vi "ChangeAssignedShortcut.vi"(7 "QDKS Info":T1[](array[typedef]), 8 "error in (no error)":errorcluster, 10 "Key":string, 11 "QD":string) -> (0 "error out":errorcluster)   [LabVIEW 2020, in "NEVSTOP QD Shortcuts.lvlib"]
uses:
  NEVSTOP QD Shortcuts.lvlib
  <resource>/dialog/QuickDrop/QuickDrop QDKS Info.ctl
  <resource>/dialog/lvconfig.llb/LV Config Write String.vi
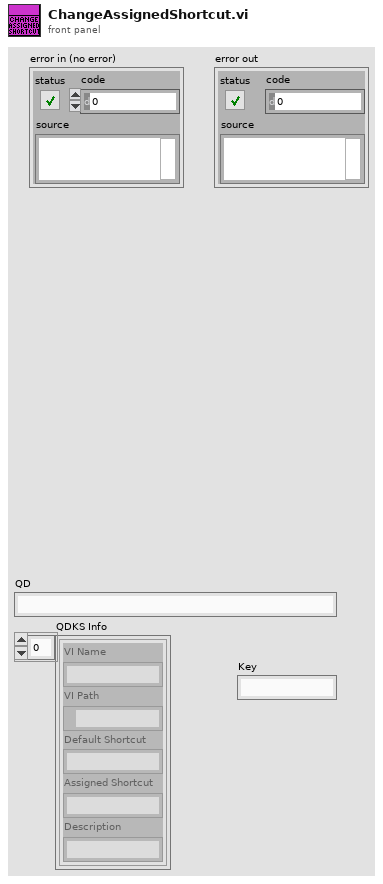
[diagram p1: front panel]
types:
  T1 = typedef "QuickDrop QDKS Info.ctl" = cluster{"VI Name":string, "VI Path":path, "Default Shortcut":string, "Assigned Shortcut":string, "Description":string}
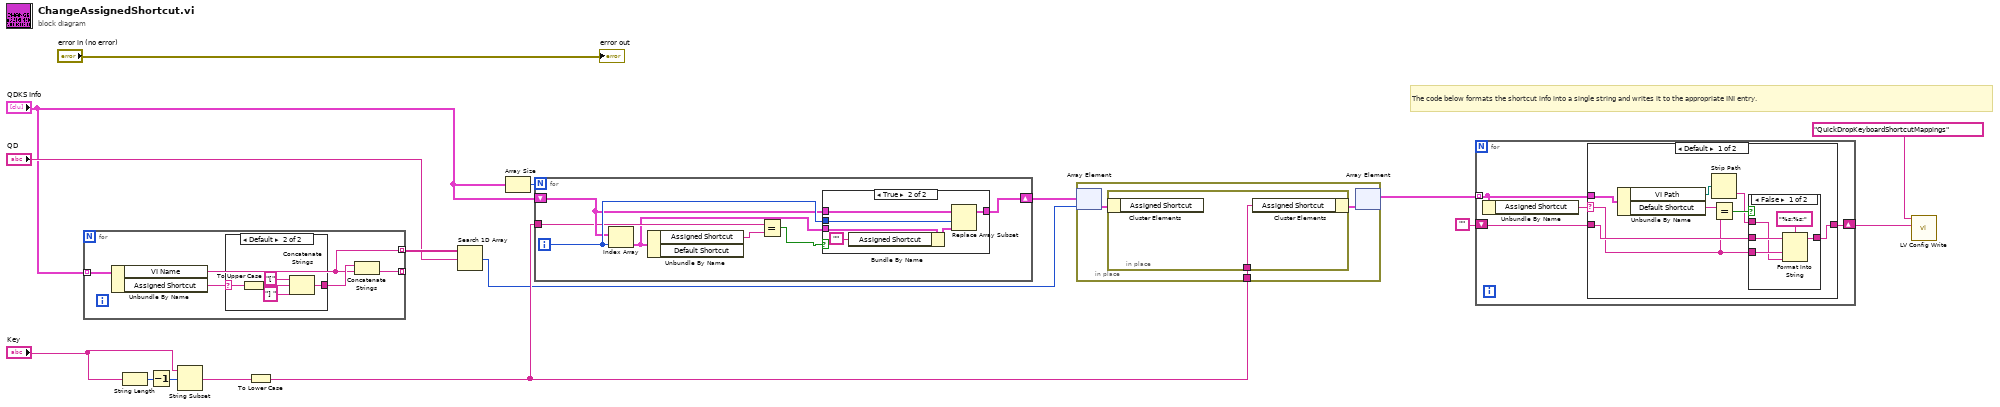
[diagram p0: block diagram]
diagram:
  # "The code below formats the shortcut info into a single string and writes it to the appropriate INI entry."
  n1 = for {
    tunnel: "QDKS Info" -> [w21] mode=indexing
    tunnel: [w20] -> _ mode=indexing
    tunnel: [w17] -> w7 mode=indexing
    n2 = Unbundle By Name(w21) -> ("VI Name"=w17:string, "Assigned Shortcut"=w19:string)
    n3 = case shown="Default" w19 {
      selector: w19 -> [_ w26]
      tunnel: [_ w25] -> w18
      frame "" {
      }
      frame Default {
        n4 = To Upper Case(1:w26) -> (0:w22:string)
        n5 = Concatenate Strings("[" ("string"), w22, "] " ("string")) -> (w25:string)
      }
    }
    n6 = Concatenate Strings(w18, w17) -> (w20:string)
  }
  n7 = String Length(string="Key") -> (length=w15:i32)
  n8 = Decrement(x=w15) -> (x-1=w14:i32)
  n9 = String Subset(string="Key", offset (0)=w14) -> (substring=w13:string)  [unwired: 1 in]
  n10 = To Lower Case(string=w13) -> (all lower case string=w11:string)
  n11 = Search 1D Array(1D array=w7, element="QD") -> (index of element=w5:i32)  [unwired: 1 in]
  n12 = Array Size(array="QDKS Info") -> (size(s)=w12:i32)
  n13 = for {
    N: w12 -> [_]
    shift-right: [w31] -> w2
    shift-left: "QDKS Info" -> [w32]
    tunnel: w11 -> [w30]
    i -> [w33]
    n14 = Index Array(array=w32, index=w33) -> (element=w28:T1)
    n15 = Unbundle By Name(w28) -> ("Assigned Shortcut"=w29:string)  [unwired: 1 out]
    n16 = Equal?(x=w30, y=w29) -> (x = y?=w27:bool)
    n17 = case shown="True" w27 {
      tunnel: w32 -> [w34 w40]
      tunnel: [w34 w39] -> w31
      tunnel: w33 -> [_ w38]
      tunnel: w28 -> [_ w37]
      frame False {
      }
      frame True {
        n18 = Bundle By Name(cluster=w37, "Assigned Shortcut"="") -> (w36:T1)
        n19 = Replace Array Subset(array=w40, new element=w36, index=w38) -> (w39:T1[])
      }
    }
  }
  n20 = in-place {
    in-place-border: w11 -> [w41]
    n21 = in-place-array #1(w2, w5) -> (w43:T1)
    n22 = in-place {
      in-place-border: w41 -> [w44]
      n23 = in-place-cluster #2(w43) -> ()  [unwired: 1 out]
      n24 = in-place-cluster #2("Assigned Shortcut"=w44) -> (w42:T1)
    }
    n25 = in-place-array #1(w42) -> (w1:T1[])  [unwired: 1 out]
  }
  n26 = for {
    tunnel: w1 -> [w45] mode=indexing
    shift-right: [w46] -> w9
    shift-left: "" -> [w47]
    n27 = Unbundle By Name(w45) -> ("Assigned Shortcut"=w48:string)
    n28 = case shown="Default" w48 {
      selector: w48 -> [w52 _]
      tunnel: w47 -> [w54 w63]
      tunnel: [w55 w63] -> w46
      tunnel: w45 -> [w56 _]
      frame Default {
        n29 = Unbundle By Name(w56) -> ("VI Path"=w50:path, "Default Shortcut"=w53:string)
        n30 = Strip Path(path=w50) -> (name=w49:string)  [unwired: 1 out]
        n31 = Equal?(x=w53, y=w52) -> (x = y?=w51:bool)
        n32 = case shown="False" w51 {
          tunnel: [w61 w62] -> w55
          tunnel: w54 -> [w59 w62]
          tunnel: w52 -> [w58 _]
          tunnel: w49 -> [w57 _]
          frame False {
            n33 = Format Into String(format string="%s:%s;", initial string=w59, w58, w57) -> (resulting string=w61:string)  [unwired: 1 in, 1 out]
          }
          frame True {
          }
        }
      }
      frame "" {
      }
    }
  }
  n34 = call-poly <resource>:"LV Config Write.vi"("value"=w9, "key"="QuickDropKeyboardShortcutMappings" ("Name")) -> ()  [unwired: 1 in, 5 out]
  "error out" <- "error in (no error)"
